vi "Depricate.vi"(8 "error in (no error)":errorcluster, 10 "Name Array":string[](array[string]), 11 "JSON Array In":refnum<class "JSON Array.lvclass">) -> (0 "error out":errorcluster, 1 "Value":refnum<class "JSON Value.lvclass">, 2 "found":bool, 3 "JSON Array Out":refnum<class "JSON Array.lvclass">)   [LabVIEW 2011]
uses:
  JSON Array.lvclass
  JSON Value/JSON Value.lvclass
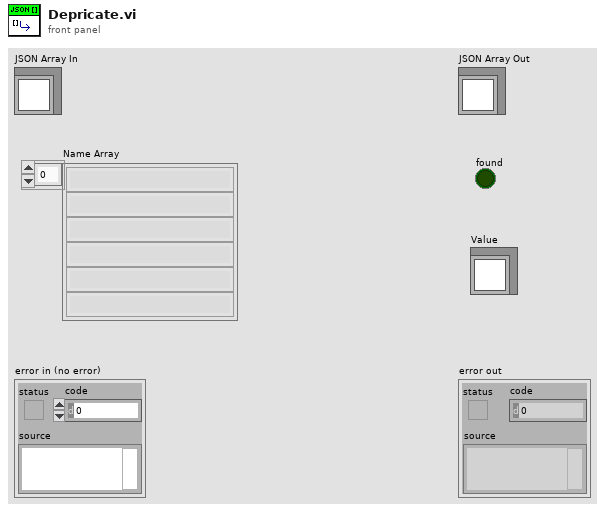
[diagram p1: front panel]
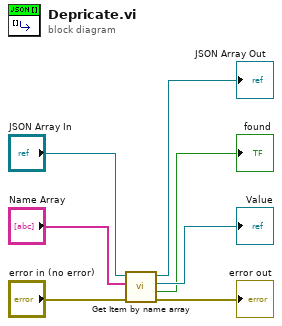
[diagram p0: block diagram]
diagram:
  n1 = call "Get Item by name array.vi"("error in (no error)"="error in (no error)", "Name Array"="Name Array", "JSON Value In"="JSON Array In") -> ("error out"=→"error out":errorcluster, "found"=→"found":bool, "Value"=→"Value":refnum<class "JSON Value.lvclass">, "JSON Value Out"=→"JSON Array Out":refnum<class "JSON Array.lvclass">)  [unwired: 5 in]
